vi "Calibration_user_input.vi"(4 "data mode":enum16{"Take new data point", "Refit Curve"}(ring), 6 "Mode":T4, 7 "Fixed n":bool, 8 "OK":T14, 9 "Sampling speeds":T5={"Samples /ch"=300, "Sampling Rate /ch (Hz)"=50.0} {"Sampling Rate /ch (Hz)" min=0 format="%.2f"; "Samples /ch" min=0 step=1}) -> (1 "Sampling speeds Output":T5={"Samples /ch"=300, "Sampling Rate /ch (Hz)"=50.0} {"Sampling Rate /ch (Hz)" min=0 format="%.2f"; "Samples /ch" min=0 step=1}, 2 "Fixed n out":bool, 3 "Temp (deg C)":dbl=21.0 format="%.1f", 5 "Abs Press (mbar)":dbl=1013.0 format="%.1f")   [LabVIEW 2011]
uses:
  Controls/ok_button.ctl
  Controls/Board_Types.ctl
  Controls/Cal_Inst_type.ctl
  Calib_setup.ctl
  Controls/Ref_Inst_type.ctl
  Calib_mode.ctl
  Controls/PWA_Data.ctl
  File/Setup_Filetype.ctl
  Controls/Inst_type.ctl
  ADAM Client/Sub VIs/ADAM Controls/Channel_names.ctl
  Controls/Setup.ctl
  Globals/Calib_global.vi
  Globals/Meas_global.vi
  Globals/LDA_meas_global_1.vi
  Globals/LDA_meas_global_2.vi
panel:
  in  "PWA Data":T1
  in  "Preston tube diammeter in mm":dbl min=0.0
  in  "Reference instrument Orig":T3={"high limit (10V)"=4.0, "low limit (-10V)"=0.0, "Ch No"=4, "Off ch no"=0, "Calib filename"=path "", "Ref Instrument type"=enum."Enter Value"} {"Off ch no" min=0 max=1; "Ch No" min=0 max=7; "low limit (-10V)" min=-10 max=10 format="%.1f"; "high limit (10V)" min=-10 max=10 format="%.1f"}
  out "Message":string
  in  "Ref Instrument type":T2
  out "Info":string
  out "XW Angle Calib Present?":bool
  out "XW Velocity Calib Present?":bool
  in  "Edit temp and Press":bool
  out "2nd ref instrument":T6={"2nd Ref type"=enum."LDA", "2nd inst present"=TRUE}
  in  "Ref vel for angle calib":T7={"high limit (10V)"=6.0, "low limit (-10V)"=0.0, "Ch No"=4, "Off ch no"=0, "Calib filename"=path "", "Ref Instrument type"=enum."LDA"} {"Off ch no" min=0 max=1; "Ch No" min=0 max=50; "low limit (-10V)" min=-10 max=10 format="%.1f"; "high limit (10V)" min=-10 max=10 format="%.1f"}
  out "Instrument type":T8=enum."Cross wire angle"
  in  "angle calib":T9(ring)
  in  "Reference instrument":T7={"high limit (10V)"=4.0, "low limit (-10V)"=0.0, "Ch No"=4, "Off ch no"=0, "Calib filename"=path "", "Ref Instrument type"=enum."Enter Value"} {"Off ch no" min=0 max=1; "Ch No" min=0 max=50; "low limit (-10V)" min=-10 max=10 format="%.1f"; "high limit (10V)" min=-10 max=10 format="%.1f"}
  in  "instrument to calibrate":T10(array[cluster])=[{"high limit (10V)"=5.0, "low limit (-10V)"=3.0, "Ch No"=1, "Off ch no"=1}, {"high limit (10V)"=5.0, "low limit (-10V)"=3.0, "Ch No"=2, "Off ch no"=1}] {"Off ch no" min=0 max=1; "Ch No" min=0 max=50; "low limit (-10V)" min=-10 max=10 format="%.3f"; "high limit (10V)" min=-10 max=10 format="%.3f"}
  in  "Instrument type":T8=enum."Pressure Transducer"
  out "Calib filename":path
  in  "Type":T11={"high limit (10V)"=4.0, "low limit (-10V)"=0.0, "Ch No"=4, "Var name"="LDA"} {"Ch No" min=0 max=7; "low limit (-10V)" min=-10 max=10 format="%.3f"; "high limit (10V)" min=-10 max=10 format="%.3f"}
  in  "Acquisition Method":T12
  out "Ch & spans":T13(array[cluster])=[{"high limit (10V)"=5.0, "low limit (-10V)"=3.0, "Ch No"=1, "Var name"="Cross wire 1"}, {"high limit (10V)"=5.0, "low limit (-10V)"=3.0, "Ch No"=2, "Var name"="Cross wire 2"}] {"Ch No" min=0 max=7; "low limit (-10V)" min=-10 max=10 format="%.3f"; "high limit (10V)" min=-10 max=10 format="%.3f"}
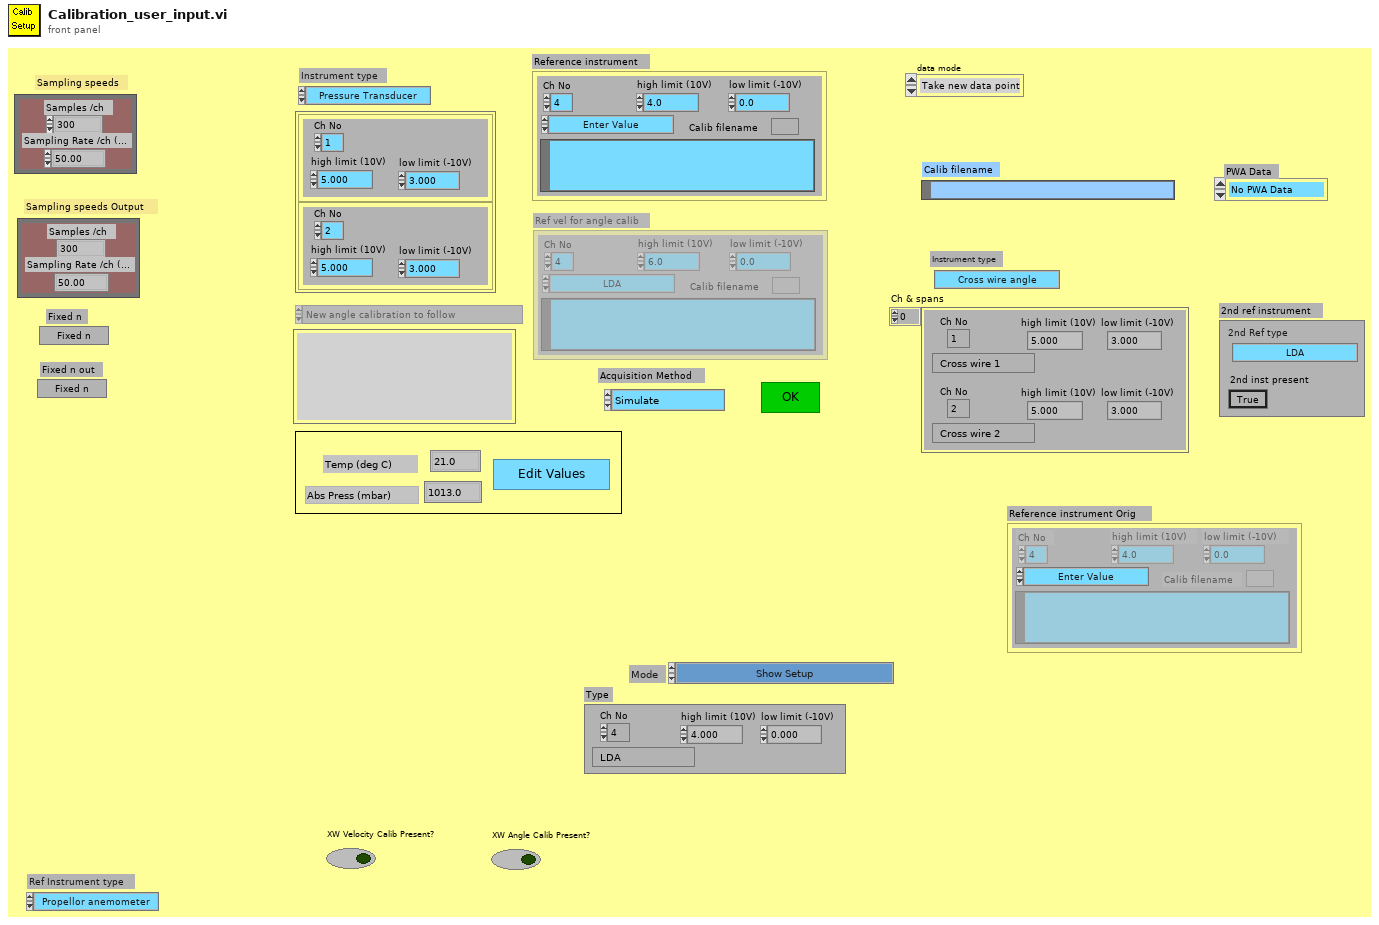
[diagram p1: front panel]
types:
  T1 = typedef "PWA_Data.ctl" = enum16{"No PWA Data", "One Ch PWA"}
  T2 = typedef "Ref_Inst_type.ctl" = enum16{"Propellor anemometer", "Pressure Transducer", "Raw voltage", "Pitot-static tube", "Preston tube", "Generic Linear", "Generic Polynomial", "Thermocouple", "LDA", "Enter Value", "ADAM Channel"}
  T3 = cluster{"high limit (10V)":sgl, "low limit (-10V)":sgl, "Ch No":i16, "Off ch no":i8, "Calib filename":path, "Ref Instrument type":T2}
  T4 = typedef "Calib_mode.ctl" = enum16{"Show Setup", "Take a New Calibration Point", "Refit Curve", "Setup Front Panel"}
  T5 = cluster{"Samples /ch":i32, "Sampling Rate /ch (Hz)":sgl}
  T6 = cluster{"2nd Ref type":T2, "2nd inst present":bool}
  T7 = typedef "Calib_setup.ctl" = cluster{"high limit (10V)":sgl, "low limit (-10V)":sgl, "Ch No":i16, "Off ch no":i8, "Calib filename":path, "Ref Instrument type":T2}
  T8 = typedef "Cal_Inst_type.ctl" = enum16{"Propeller anemometer", "Pressure Transducer", "Hot wire", "Cross wire velocity", "Cross wire angle", "Generic Linear", "Generic Polynomial", "Generic BackPoly", "Fast FID", "Thermocouple", "Cold wire", "Pulsed Wire"}
  T9 = enum16{"New angle calibration to follow", "Use the most recent angle calibration"}
  T10 = cluster{"high limit (10V)":sgl, "low limit (-10V)":sgl, "Ch No":i16, "Off ch no":i8}[]
  T11 = cluster{"high limit (10V)":sgl, "low limit (-10V)":sgl, "Ch No":i16, "Var name":string}
  T12 = typedef "Board_Types.ctl" = enum16{"Simulate", "Local ADAM", "Server ADAM", "NI-DAQmx", "NI-DAQmxBase", "ADC488", "DT LV-link"}
  T13 = cluster{"high limit (10V)":sgl, "low limit (-10V)":sgl, "Ch No":i16, "Var name":string}[]
  T14 = typedef "ok_button.ctl" = bool
  T15 = typedef "Setup_Filetype.ctl" = enum16{"Measurement Setups", "Calibration Setups", "General", "Results File Plotter Setups", "Speed Calib Tweaks"}
  T16 = typedef "Inst_type.ctl" = enum16{"Propeller anemometer", "Raw voltage", "Pressure Transducer", "Pitot-static tube", "Preston tube", "Hot wire", "Cross wire 1", "Cross wire 2", "Generic Linear", "Generic Polynomial", "Generic BackPoly", "Fast FID", "Thermocouple", "Cold wire", "Pulsed Wire", "LDA Vel", "LDA Tran time", "LDA Arr time"}
  T17 = typedef "Channel_names.ctl" = enum16{"Active Only", "Active + Off", "All Channels"}
  T18 = typedef "Setup.ctl" = enum16{"Run Program", "Show Setup", "Save Current Setup", "Setup Front Panel"}
  T19 = cluster{"high limit (10V)":sgl, "low limit (-10V)":sgl, "Ch No":i16, "Off ch no":i8}
  T20 = typedef "BSA_Type.ctl" = enum16{"57N11", "BSA F60"}
  T21 = typedef "BSA_info_Cluster.ctl" = cluster{"GPIB Address":string, "No of Check Bytes":i32, "Extra Info":string, "COLOUR":u32, "Wavelength (nm)":dbl}
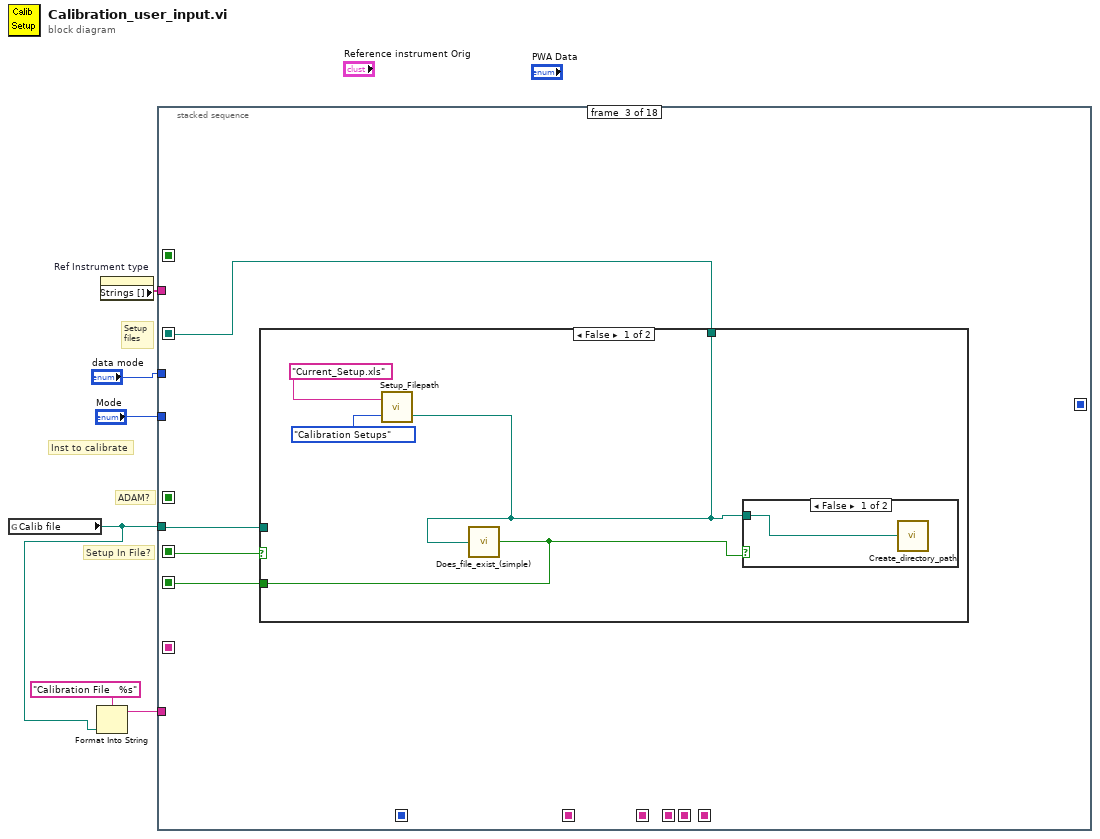
[diagram p0: block diagram]
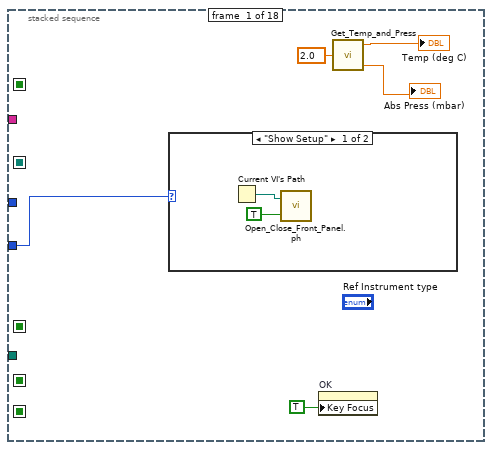
[diagram p2: hidden frame]
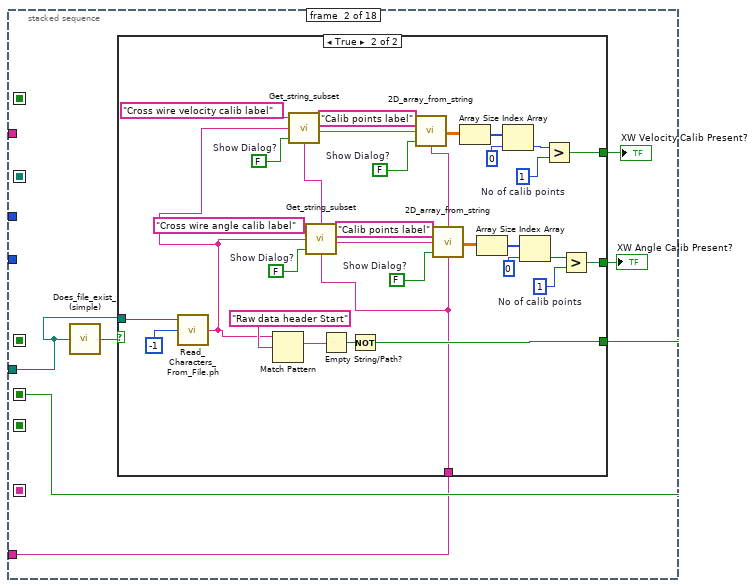
[diagram p4: hidden frame]
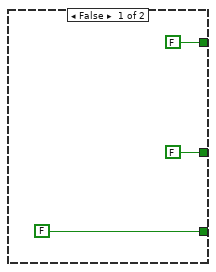
[diagram p5: hidden frame]
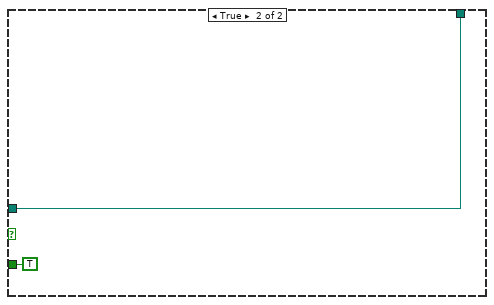
[diagram p7: hidden frame]
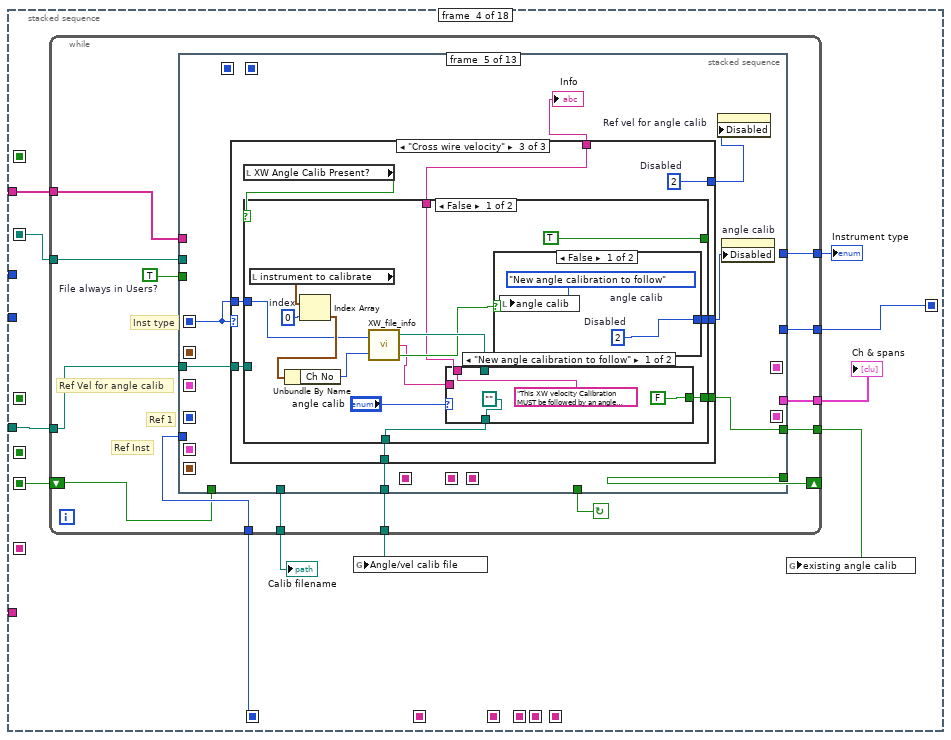
[diagram p8: hidden frame]
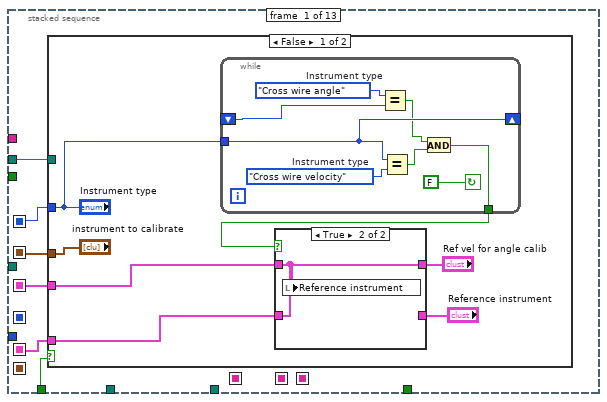
[diagram p9: hidden frame]
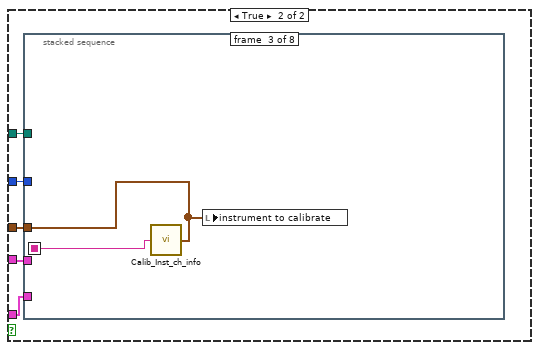
[diagram p11: hidden frame]
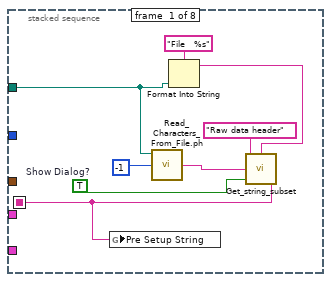
[diagram p12: hidden frame]
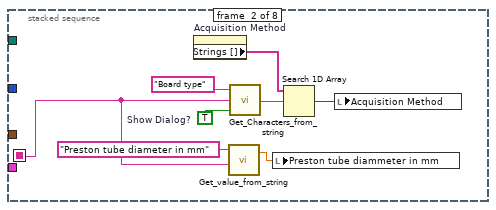
[diagram p13: hidden frame]
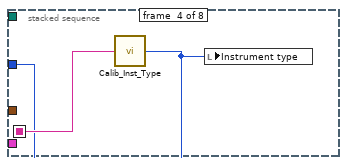
[diagram p14: hidden frame]
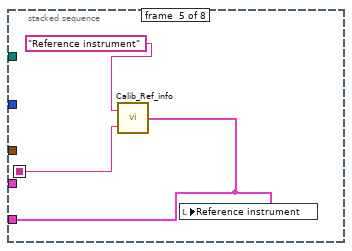
[diagram p15: hidden frame]
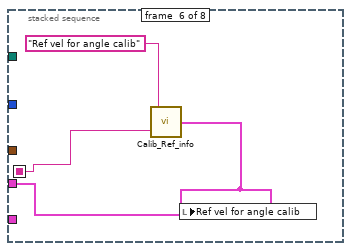
[diagram p16: hidden frame]
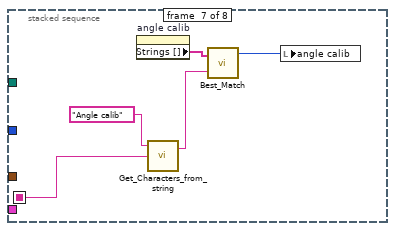
[diagram p17: hidden frame]
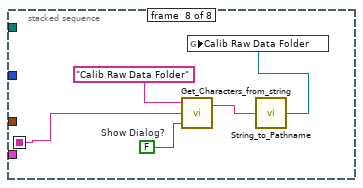
[diagram p18: hidden frame]
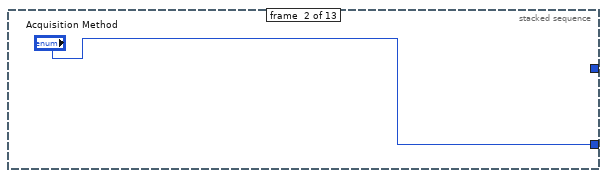
[diagram p19: hidden frame]
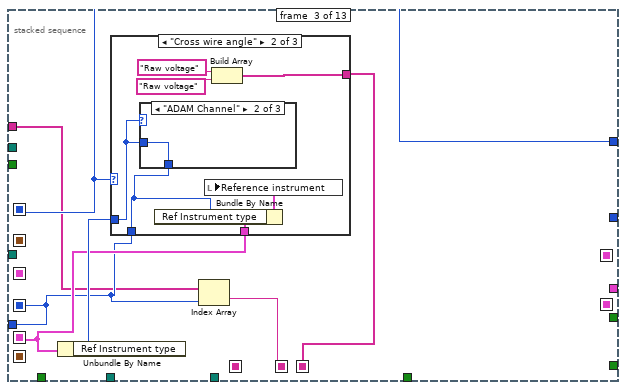
[diagram p20: hidden frame]
diagram:
  # "Inst to calibrate"
  # "Setup In File?"
  # "Setup\nfiles"
  # "ADAM?"
  n1 = global read "Calib_global.vi" "Calib file"() -> (w2:path)
  n2 = Format Into String(format string="Calibration File   %s", w2) -> (resulting string=w1:string)  [unwired: 2 in, 1 out]
  n3 = property on="Ref Instrument type" class="Enum (strict)"() -> ("Strings []"=w4:string[])  [unwired: 2 in, 2 out]
  n4 = stacked-sequence {
    seq-local: [_ _ w55 _ _ _ _ _ _ _ _ _ _ _ _ _ _ _] -> [_ _ _ w72 _ _ _ _ _ _ _ _ _ _ _ _ _ _]
    seq-local: [_ _ w56 _ _ _ _ _ _ _ _ _ _ _ _ _ _ _] -> [_ _ _ w70 _ _ _ _ _ _ _ _ _ _ _ _ _ _]
    seq-local: [_ _ _ w69 _ _ _ _ _ _ _ _ _ _ _ _ _ _] -> [_ _ _ _ _ _ _ w603 _ _ _ _ _ _ _ _ _ _]
    seq-local: [_ _ _ _ _ _ _ w604 _ _ _ _ _ _ _ _ _ _] -> [_ _ _ _ _ _ _ _ w621 _ _ _ _ _ _ _ _ _]
    seq-local: [_ _ _ _ _ _ _ _ w624 _ _ _ _ _ _ _ _ _] -> [_ _ _ _ _ _ _ _ _ _ _ _ _ _ w801 _ _ _]
    seq-local: [_ _ _ w68 _ _ _ _ _ _ _ _ _ _ _ _ _ _] -> [_ _ _ _ _ _ _ _ _ _ w716 _ _ _ _ _ _ _]
    seq-local: [_ _ _ _ _ _ _ _ _ _ w713 _ _ _ _ _ _ _] -> [_ _ _ _ _ _ _ _ _ _ _ _ _ _ w800 _ w835 _]
    seq-local: [_ _ _ _ _ _ _ _ _ _ w710 _ _ _ _ _ _ _] -> [_ _ _ _ _ _ _ _ _ _ _ _ _ _ _ w807 _ _]
    seq-local: [_ w19 _ _ _ _ _ _ _ _ _ _ _ _ _ _ _ _] -> [_ _ w54 _ _ _ _ _ _ _ _ _ _ _ _ _ _ _]
    seq-local: [_ _ _ _ _ _ _ _ _ _ _ w726 _ _ _ _ _ _] -> [_ _ _ _ _ _ _ _ _ _ _ _ _ _ w793 _ _ _]
    seq-local: [_ _ _ _ _ _ _ _ _ _ _ _ _ w751 _ _ _ _] -> [_ _ _ _ _ _ _ _ _ _ _ _ _ _ w781 _ _ _]
    seq-local: [_ _ _ _ _ _ _ _ _ _ _ _ w733 _ _ _ _ _] -> [_ _ _ _ _ _ _ _ _ _ _ _ _ _ w777 _ w825 _]
    seq-local: [_ _ _ _ _ _ _ _ _ w659 _ _ _ _ _ _ _ _] -> [_ _ _ _ _ _ _ _ _ _ _ _ _ _ w776 _ _ _]
    tunnel: "Mode" -> [w7 _ _ _ w526 w544 _ _ w623 w672 _ _ w734 _ _ w809 _ w852]
    tunnel: "data mode" -> [_ _ _ _ w520 _ _ _ _ _ _ _ _ _ _ _ _ _]
    tunnel: w2 -> [_ w17 w53 w65 _ _ _ _ _ _ _ _ _ _ _ _ _ _]
    tunnel: w4 -> [_ _ _ w64 _ _ _ _ _ _ _ _ _ _ _ _ _ _]
    tunnel: w1 -> [_ w14 _ _ _ _ _ _ _ _ _ _ _ _ _ _ _ _]
    frame #0 {
      n5 = case shown="\"Show Setup\"" w7 {
        frame "Show Setup" {
          n6 = Current VI's Path() -> (path=w13:path)
          n7 = call "Open_Close_Front_Panel.ph.vi"("Front Panel Window:Open"=TRUE, "VI path"=w13) -> ()  [unwired: 2 out]
        }
        frame "Take a New Calibration Point", Default {
        }
      }
      n8 = property on="OK" class="Bool"("Key Focus"=TRUE) -> ()  [unwired: 2 in, 2 out]
      n9 = call "Get_Temp_and_Press.vi"("Averaging time (mins)"=2.0) -> ("Abs Press (mbar)"=→"Abs Press (mbar)":dbl, "Temperature"=→"Temp (deg C)":dbl)  [unwired: 3 out]
    }
    frame #1 {
      n10 = call "Does_file_exist_(simple).vi"("Pathname"=w17) -> ("exists?"=w18:bool)
      n11 = case shown="True" w18 {
        tunnel: [FALSE w48] -> w19
        tunnel: w17 -> [_ w47]
        tunnel: [FALSE w25] -> w16
        tunnel: [FALSE w24] -> w15
        tunnel: w14 -> [_ w23]
        frame False {
        }
        frame True {
          w36 = 1  # No of calib points
          w30 = FALSE  # Show Dialog?
          w28 = FALSE  # Show Dialog?
          w37 = 1  # No of calib points
          w43 = FALSE  # Show Dialog?
          w45 = FALSE  # Show Dialog?
          n12 = call "Read_Characters_From_File.ph.vi"("file path (dialog if empty)"=w47, "number of characters (all:-1)"=-1) -> ("character string"=w26:string)  [unwired: 7 out]
          n13 = Match Pattern(string=w26, regular expression="Raw data header Start") -> (match substring=w50:string)  [unwired: 4 out]
          n14 = call "Get_string_subset.vi"("String Name"=w23, "Show Dialog?"=w28, "String to split"=w26, "File Label"="Cross wire velocity calib label") -> ("Output string"=w34:string)  [unwired: 1 out]
          n15 = call "Get_string_subset.vi"("String Name"=w23, "Show Dialog?"=w45, "String to split"=w26, "File Label"="Cross wire angle calib label") -> ("Output string"=w39:string)  [unwired: 1 out]
          n16 = Empty String/Path?(string/path=w50) -> (empty?=w49:bool)
          n17 = Not(x=w49) -> (.not. x?=w48:bool)
          n18 = call "2D_array_from_string.vi"("String Name"=w23, "Show Dialog?"=w30, "Input string"=w34, "Array title"="Calib points label") -> ("2D data array"=w31:dbl[][])
          n19 = call "2D_array_from_string.vi"("String Name"=w23, "Show Dialog?"=w43, "Input string"=w39, "Array title"="Calib points label") -> ("2D data array"=w42:dbl[][])
          n20 = Array Size(array=w31) -> (size(s)=w32:i32[])
          n21 = Array Size(array=w42) -> (size(s)=w41:i32[])
          n22 = Index Array(array=w32, index=0 ("Index")) -> (element=w35:i32)
          n23 = Index Array(array=w41, index=0 ("Index")) -> (element=w38:i32)
          n24 = Greater?(x=w35, y=w36) -> (0:w24:bool)
          n25 = Greater?(x=w38, y=w37) -> (0:w25:bool)
        }
      }
      "XW Velocity Calib Present?" <- w15
      "XW Angle Calib Present?" <- w16
    }
    frame #2 {
      n26 = case shown="False" w54 {
        tunnel: [w60 TRUE ("exists")] -> w56
        tunnel: [w57 w63] -> w55
        tunnel: w53 -> [_ w63]
        frame False {
          n27 = call "Setup_Filepath.vi"("Setup File Type"=Setup_Filetype."Calibration Setups", "Filename in"="Current_Setup.xls") -> ("Filename Out"=w57:path)  [unwired: 1 out]
          n28 = call "Does_file_exist_(simple).vi"("Pathname"=w57) -> ("exists?"=w60:bool)
          n29 = case shown="False" w60 {
            tunnel: w57 -> [w61 _]
            frame False {
              n30 = call "Create_directory_path.vi"("Path name"=w61) -> ()  [unwired: 1 in, 2 out]
            }
            frame True {
            }
          }
        }
        frame True {
        }
      }
    }
    frame #3 {
      n31 = while {
        tunnel: w64 -> [w78]
        shift-left: w70 -> [w81]
        shift-right: [w80] -> _
        tunnel: [w82] -> w71
        tunnel: w72 -> [w83]
        tunnel: [w84] -> w67
        tunnel: [w85] -> w74
        tunnel: [w86] -> w69
        tunnel: [w87] -> w73
        tunnel: [w88] -> w68
        tunnel: [w76] -> w66
        tunnel: w65 -> [w75]
        stop <- w79 continue-if-true
        w77 = TRUE  # File always in Users?
        # "Ref 1"
        # "Ref Inst"
        # "Ref Vel for angle calib"
        # "Inst type"
        n32 = stacked-sequence {
          seq-local: [_ _ w157 _ _ _ _ _ _ _ _ _ _] -> [_ _ _ _ _ w273 _ _ _ _ _ _ _]
          seq-local: [_ _ w161 _ _ _ _ _ _ _ _ _ _] -> [_ _ _ _ _ _ _ _ w424 _ _ _ _]
          seq-local: [_ _ _ _ _ w267 _ _ _ _ _ _ _] -> [_ _ _ _ _ _ _ _ _ w441 _ _ _]
          seq-local: [_ _ w156 _ _ _ _ _ _ _ _ _ _] -> [_ _ _ _ _ _ _ _ _ w439 _ _ _]
          seq-local: [_ _ _ _ _ _ _ _ w423 _ _ _ _] -> [_ _ _ _ _ _ _ _ _ w440 _ _ _]
          seq-local: [_ _ _ _ _ _ _ w345 _ _ _ _ _] -> [_ _ _ _ _ _ _ _ _ w436 _ _ _]
          seq-local: [_ _ _ _ _ _ w341 _ _ _ _ _ _] -> [_ _ _ _ _ _ _ _ _ w435 _ _ _]
          seq-local: [w92 _ _ _ _ _ _ _ _ _ _ _ _] -> [_ _ w159 w184 w197 _ _ w346 _ _ _ _ _]
          seq-local: [w91 _ _ _ _ _ _ _ _ _ _ _ _] -> [_ _ _ w183 _ _ _ _ _ _ _ _ _]
          seq-local: [w90 _ _ _ _ _ _ _ _ _ _ _ _] -> [_ _ _ _ _ _ w343 w347 _ w434 _ _ _]
          seq-local: [w89 _ _ _ _ _ _ _ _ _ _ _ _] -> [_ _ w158 _ _ _ _ _ _ w433 _ _ w519]
          seq-local: [_ _ _ _ _ _ _ _ _ w432 _ _ _] -> [_ _ _ _ _ _ _ _ _ _ _ w478 _]
          seq-local: [_ _ _ w179 _ _ _ _ _ _ _ _ _] -> [_ _ _ _ _ _ _ _ w422 _ _ _ _]
          tunnel: [_ "Acquisition Method" _ _ _ _ _ _ _ _ _ _ _] -> w88
          tunnel: [_ _ _ _ _ _ _ _ _ w438 _ _ _] -> w87
          tunnel: [_ _ w157 _ _ _ _ _ _ _ _ _ _] -> w86
          tunnel: [_ _ _ _ _ _ _ _ _ w432 _ _ _] -> w85
          tunnel: [_ _ _ _ w202 _ _ _ _ _ _ _ _] -> w84
          tunnel: w83 -> [w94 _ _ _ _ _ _ _ _ _ _ _ _]
          tunnel: [_ _ w159 _ _ _ _ _ _ _ _ _ _] -> w82
          tunnel: w81 -> [w93 _ _ _ _ _ _ _ _ _ _ _ _]
          tunnel: [_ _ _ _ _ _ _ _ _ _ _ FALSE _] -> w80
          tunnel: [_ _ _ _ _ _ _ _ _ _ _ w476 _] -> w79
          tunnel: w78 -> [_ _ w155 _ _ _ w340 _ _ _ _ _ _]
          tunnel: w77 -> [_ _ _ _ _ _ _ _ _ _ _ _ _]
          tunnel: [_ _ _ _ w201 _ _ _ _ _ _ _ _] -> w76
          tunnel: w75 -> [_ _ _ _ w203 _ _ _ _ _ _ _ _]
          frame #0 {
            n33 = case shown="False" w93 {
              tunnel: w94 -> [_ w117]
              tunnel: ["Instrument type" w115] -> w92
              tunnel: ["instrument to calibrate" w116] -> w91
              tunnel: [w96 w113] -> w90
              tunnel: [w98 w114] -> w89
              frame False {
                n34 = while {
                  shift-right: [w110] -> _
                  shift-left: _ -> [w108]
                  tunnel: "Instrument type" -> [w110]
                  tunnel: [w105] -> w99
                  stop <- FALSE continue-if-true
                  w109 = Cal_Inst_type."Cross wire angle"  # Instrument type
                  w111 = Cal_Inst_type."Cross wire velocity"  # Instrument type
                  n35 = Equal?(x=w109, y=w108) -> (x = y?=w106:bool)
                  n36 = Equal?(x=w110, y=w111) -> (x = y?=w107:bool)
                  n37 = And(x=w106, y=w107) -> (x .and. y?=w105:bool)
                }
                n38 = case shown="True" w99 {
                  tunnel: [w103 w104] -> w98
                  tunnel: "Reference instrument" -> [w103 _]
                  tunnel: [w102 w104] -> w96
                  tunnel: "Ref vel for angle calib" -> [w102 w104]
                  frame False {
                  }
                  frame True {
                    n39 = local write "Reference instrument"(w104) -> ()
                  }
                }
              }
              frame True {
                n40 = stacked-sequence {
                  seq-local: [w122 _ _ _ _ _ _ _] -> [_ w128 w135 w137 w139 w142 w146 w151]
                  tunnel: w117 -> [w119 _ _ _ _ _ _ _]
                  tunnel: [_ _ w134 _ _ _ _ _] -> w116
                  tunnel: [_ _ _ w136 _ _ _ _] -> w115
                  tunnel: [_ _ _ _ w138 _ _ _] -> w114
                  tunnel: [_ _ _ _ _ w141 _ _] -> w113
                  frame #0 {
                    w121 = TRUE  # Show Dialog?
                    n41 = call "Read_Characters_From_File.ph.vi"("file path (dialog if empty)"=w119, "number of characters (all:-1)"=-1) -> ("character string"=w125:string)  [unwired: 7 out]
                    n42 = Format Into String(format string="File   %s", w119) -> (resulting string=w118:string)  [unwired: 2 in, 1 out]
                    n43 = call "Get_string_subset.vi"("String Name"=w118, "Show Dialog?"=w121, "String to split"=w125, "File Label"="Raw data header") -> ("Output string"=w122:string)  [unwired: 1 out]
                    n44 = global write "Calib_global.vi" "Pre Setup String"(w122) -> ()
                  }
                  frame #1 {
                    w133 = TRUE  # Show Dialog?
                    n45 = property on="Acquisition Method" class="Enum (strict)"() -> ("Strings []"=w129:string[])  [unwired: 2 in, 2 out]
                    n46 = call "Get_value_from_string.vi"("Input string"=w128, "Variable name"="Preston tube diameter in mm") -> ("Value"=w126:dbl)  [unwired: 1 in, 1 out]
                    n47 = call "Get_Characters_from_string.vi"("Show Dialog?"=w133, "Input string"=w128, "Variable name"="Board type") -> ("Value"=w131:string)  [unwired: 1 out]
                    n48 = local write "Preston tube diammeter in mm"(w126) -> ()
                    n49 = Search 1D Array(1D array=w129, element=w131) -> (index of element=w130:i32)  [unwired: 1 out]
                    n50 = local write "Acquisition Method"(w130) -> ()
                  }
                  frame #2 {
                    n51 = call "Calib_Inst_ch_info.vi"("Input string"=w135) -> ("instrument to calibrate"=w134:T10)
                    n52 = local write "instrument to calibrate"(w134) -> ()
                  }
                  frame #3 {
                    n53 = call "Calib_Inst_Type.vi"("Input string"=w137) -> ("Instrument type"=w136:T8)
                    n54 = local write "Instrument type"(w136) -> ()
                  }
                  frame #4 {
                    n55 = call "Calib_Ref_info.vi"("Input string"=w139, "Reference Name"="Reference instrument") -> ("Reference instrument"=w138:T7)
                    n56 = local write "Reference instrument"(w138) -> ()
                  }
                  frame #5 {
                    n57 = call "Calib_Ref_info.vi"("Input string"=w142, "Reference Name"="Ref vel for angle calib") -> ("Reference instrument"=w141:T7)
                    n58 = local write "Ref vel for angle calib"(w141) -> ()
                  }
                  frame #6 {
                    n59 = property on="angle calib" class="Enum (strict)"() -> ("Strings []"=w148:string[])  [unwired: 2 in, 2 out]
                    n60 = call "Get_Characters_from_string.vi"("Input string"=w146, "Variable name"="Angle calib") -> ("Value"=w145:string)  [unwired: 1 in, 1 out]
                    n61 = call "Best_Match.vi"("Input String"=w145, "String Options"=w148) -> ("index of element"=w144:i32)  [unwired: 1 out]
                    n62 = local write "angle calib"(w144) -> ()
                  }
                  frame #7 {
                    w152 = FALSE  # Show Dialog?
                    n63 = call "Get_Characters_from_string.vi"("Show Dialog?"=w152, "Input string"=w151, "Variable name"="Calib Raw Data Folder") -> ("Value"=w150:string)  [unwired: 1 out]
                    n64 = call "String_to_Pathname.vi"("Input String"=w150) -> ("path"=w149:path)
                    n65 = global write "Calib_global.vi" "Calib Raw Data Folder"(w149) -> ()
                  }
                }
              }
            }
          }
          frame #1 {
          }
          frame #2 {
            n66 = Unbundle By Name(w158) -> ("Ref Instrument type"=w160:T2)
            n67 = case shown="\"Cross wire angle\"" w159 {
              tunnel: [w164 w172 w177] -> w161
              tunnel: w160 -> [w162 w166 w176]
              tunnel: [w162 w169 w176] -> w157
              tunnel: w158 -> [_ w170 _]
              frame "Cross wire velocity" {
                n68 = Build Array("Raw voltage", "Raw voltage") -> (w164:string[])
              }
              frame "Cross wire angle" {
                n69 = case shown="\"ADAM Channel\"" w166 {
                  tunnel: [w173 w174 Ref_Inst_type."Enter Value" ("Ref Instrument type")] -> w169
                  tunnel: w166 -> [w173 w174 _]
                  frame "Enter Value" {
                  }
                  frame "ADAM Channel" {
                  }
                  frame "LDA", Default {
                  }
                }
                n70 = Bundle By Name(cluster=w170, "Ref Instrument type"=w169) -> (w171:T7)
                n71 = local write "Reference instrument"(w171) -> ()
                n72 = Build Array("Raw voltage", "Raw voltage") -> (w172:string[])
              }
              frame "Generic Linear", Default {
                n73 = Build Array("Raw voltage") -> (w177:string[])
              }
            }
            n74 = Index Array(array=w155, index=w157) -> (element=w156:string)
          }
          frame #3 {
            n75 = Array Size(array=w183) -> (size(s)=w182:i32)
            n76 = case shown="\"Pulsed Wire\"" w184 {
              tunnel: [2 2 1 0] -> w181
              frame "Cross wire velocity" {
              }
              frame "Cross wire angle" {
              }
              frame "Generic Linear", Default {
              }
              frame "Pulsed Wire" {
              }
            }
            n77 = Equal?(x=w181, y=w182) -> (x = y?=w180:bool)
            n78 = case shown="False" w180 {
              tunnel: w181 -> [w190 _]
              tunnel: w183 -> [w186 w192]
              tunnel: [w185 w192] -> w179
              frame False {
                n79 = Index Array(array=w186, index=0) -> (element=w187:T19)
                n80 = Build Array (concatenate)(w186, w187) -> (w189:T10)
                n81 = for {
                  N: w190 -> [_]
                  tunnel: w189 -> [w191] mode=indexing
                  tunnel: [w191] -> w185 mode=indexing
                }
                n82 = local write "instrument to calibrate"(w185) -> ()
              }
              frame True {
              }
            }
          }
          frame #4 {
            n83 = case shown="\"Cross wire velocity\"" w197 {
              tunnel: w203 -> [_ w214 w236]
              tunnel: [path "" w215 w237] -> w202
              tunnel: [FALSE w213 w235] -> w201
              tunnel: [w204 w209 w231] -> w200
              tunnel: [w206 w212 w234] -> w199
              tunnel: ["" w211 w232] -> w198
              tunnel: w197 -> [_ w210 w233]
              frame "Propeller anemometer", Default {
                w204 = u8 2  # Disabled
                w206 = u8 2  # Disabled
              }
              frame "Cross wire angle" {
                w209 = u8 0  # Disabled
                w212 = u8 2  # Disabled
                n84 = local read "XW Velocity Calib Present?"() -> (w216:bool)
                n85 = case shown="False" w216 {
                  tunnel: [w220 w230] -> w215
                  tunnel: w214 -> [_ w230]
                  tunnel: [TRUE TRUE] -> w213
                  tunnel: [w218 w228] -> w211
                  tunnel: w210 -> [w217 _]
                  frame False {
                    w224 = 0  # index
                    n86 = local read "instrument to calibrate"() -> (w225:T10)
                    n87 = Index Array(array=w225, index=w224) -> (element=w223:T19)
                    n88 = Unbundle By Name(w223) -> ("Ch No"=w221:i16)
                    n89 = call "XW_file_info.vi"("Instrument type"=w217, "Ch No"=w221) -> ("Filename"=w220:path, "resulting string"=w218:string, "File Exists?"=w219:bool)
                    n90 = case shown="False" w219 {
                      frame False {
                        w226 = Cal_Inst_type."Cross wire velocity"  # Instrument type
                        w227 = "You need to do a velocity calibration before you can do the angle calibration"  # message
                        n91 = local write "Instrument type"(w226) -> ()
                        n92 = One Button Dialog(message=w227) -> ()  [unwired: 2 out]
                      }
                      frame True {
                      }
                    }
                  }
                  frame True {
                    w228 = "Will use the velocity Calibration info already in the Calibration file. "  # resulting string
                  }
                }
              }
              frame "Cross wire velocity" {
                w231 = u8 2  # Disabled
                n93 = local read "XW Angle Calib Present?"() -> (w238:bool)
                n94 = case shown="False" w238 {
                  tunnel: [w247 w266] -> w237
                  tunnel: w236 -> [_ w266]
                  tunnel: [TRUE FALSE] -> _
                  tunnel: [w246 TRUE] -> w235
                  tunnel: [w245 w263] -> w234
                  tunnel: w233 -> [w243 _]
                  tunnel: [w240 w262] -> w232
                  frame False {
                    w251 = 0  # index
                    n95 = local read "instrument to calibrate"() -> (w252:T10)
                    n96 = Index Array(array=w252, index=w251) -> (element=w250:T19)
                    n97 = Unbundle By Name(w250) -> ("Ch No"=w244:i16)
                    n98 = call "XW_file_info.vi"("Instrument type"=w243, "Ch No"=w244) -> ("Filename"=w242:path, "resulting string"=w239:string, "File Exists?"=w241:bool)
                    n99 = case shown="\"New angle calibration to follow\"" "angle calib" {
                      tunnel: [path "" w258] -> w247
                      tunnel: w242 -> [_ w258]
                      tunnel: [FALSE TRUE] -> w246
                      tunnel: ["This XW velocity Calibration MUST be followed by an angle calibration, before XW measurements can be made." w256] -> w240
                      tunnel: w239 -> [_ w256]
                      frame "New angle calibration to follow" {
                      }
                      frame "Use the most recent angle calibration" {
                      }
                    }
                    n100 = case shown="False" w241 {
                      tunnel: [w259 w261] -> w245
                      frame False {
                        w259 = u8 2  # Disabled
                        w260 = T9."New angle calibration to follow"  # angle calib
                        n101 = local write "angle calib"(w260) -> ()
                      }
                      frame True {
                        w261 = u8 0  # Disabled
                      }
                    }
                  }
                  frame True {
                    w262 = "Will use the angle Calibration info already in the Calibration file. "  # resulting string
                    w263 = u8 0  # Disabled
                  }
                }
              }
            }
            "Info" <- w198
            n102 = property on="Ref vel for angle calib" class="Clust (strict)"("Disabled"=w200) -> ()  [unwired: 2 in, 2 out]
            n103 = property on="angle calib" class="Enum (strict)"("Disabled"=w199) -> ()  [unwired: 2 in, 2 out]
          }
          frame #5 {
            n104 = case shown="\"Generic Polynomial\"" w273 {
              tunnel: [u8 0 u8 0 u8 0 u8 0 u8 0 u8 0 u8 0 u8 2 u8 2 u8 2 u8 2] -> w268
              tunnel: [u8 0 u8 0 u8 2 u8 0 u8 0 u8 0 u8 0 u8 2 u8 2 u8 2 u8 2] -> w272
              tunnel: [u8 0 u8 0 u8 0 u8 0 u8 0 u8 0 u8 0 u8 2 u8 2 u8 2 u8 2] -> w271
              tunnel: [u8 0 u8 0 u8 0 u8 0 u8 0 u8 0 u8 0 u8 2 u8 2 u8 2 u8 2] -> w270
              tunnel: [u8 0 u8 0 u8 0 u8 0 u8 0 u8 0 u8 0 u8 2 u8 2 u8 2 u8 2] -> w269
              tunnel: [1 1 1 1 1 1 1 0 0 0 0] -> w267
              frame "Propellor anemometer" {
              }
              frame "Pressure Transducer" {
              }
              frame "Raw voltage" {
              }
              frame "Pitot-static tube" {
              }
              frame "Preston tube" {
              }
              frame "Generic Linear" {
              }
              frame "Generic Polynomial" {
              }
              frame "Thermocouple" {
              }
              frame "LDA" {
              }
              frame "Enter Value" {
              }
              frame "ADAM Channel" {
              }
            }
            n105 = property on="Calib filename" class="Path"("Disabled"=w272) -> ()  [unwired: 2 in, 2 out]
            n106 = property on="Ch No" class="DigNum (strict)"("Disabled"=w271) -> ()  [unwired: 2 in, 2 out]
            n107 = property on="high limit (10V)" class="DigNum (strict)"("Disabled"=w270) -> ()  [unwired: 2 in, 2 out]
            n108 = property on="low limit (-10V)" class="DigNum (strict)"("Disabled"=w269) -> ()  [unwired: 2 in, 2 out]
            n109 = property on="Off ch no" class="DigNum (strict)"("Disabled"=w268) -> ()  [unwired: 2 in, 2 out]
          }
          frame #6 {
            n110 = Unbundle By Name(w343) -> ("Ref Instrument type"=w342:T2)
            n111 = Index Array(array=w340, index=w342) -> (element=w341:string)
          }
          frame #7 {
            n112 = Unbundle By Name(w347) -> ("Ref Instrument type"=w348:T2)
            n113 = case shown="\"Generic Polynomial\"" w348 {
              tunnel: [u8 0 u8 0 u8 0 u8 0 u8 0 u8 0 u8 0 u8 0 u8 2 u8 2 u8 2] -> w349
              tunnel: [u8 0 u8 0 u8 2 u8 0 u8 0 u8 0 u8 0 u8 0 u8 2 u8 2 u8 2] -> w353
              tunnel: [u8 0 u8 0 u8 0 u8 0 u8 0 u8 0 u8 0 u8 0 u8 2 u8 2 u8 2] -> w352
              tunnel: [u8 0 u8 0 u8 0 u8 0 u8 0 u8 0 u8 0 u8 0 u8 2 u8 2 u8 2] -> w351
              tunnel: [u8 0 u8 0 u8 0 u8 0 u8 0 u8 0 u8 0 u8 0 u8 2 u8 2 u8 2] -> w350
              tunnel: [enum16{"No 2nd ref inst", "Add 2nd ref inst"}."Add 2nd ref inst" enum16{"No 2nd ref inst", "Add 2nd ref inst"}."Add 2nd ref inst" enum16{"No 2nd ref inst", "Add 2nd ref inst"}."Add 2nd ref inst" enum16{"No 2nd ref inst", "Add 2nd ref inst"}."Add 2nd ref inst" enum16{"No 2nd ref inst", "Add 2nd ref inst"}."Add 2nd ref inst" enum16{"No 2nd ref inst", "Add 2nd ref inst"}."Add 2nd ref inst" enum16{"No 2nd ref inst", "Add 2nd ref inst"}."Add 2nd ref inst" enum16{"No 2nd ref inst", "Add 2nd ref inst"}."Add 2nd ref inst" enum16{"No 2nd ref inst", "Add 2nd ref inst"}."No 2nd ref inst" enum16{"No 2nd ref inst", "Add 2nd ref inst"}."No 2nd ref inst" enum16{"No 2nd ref inst", "Add 2nd ref inst"}."No 2nd ref inst"] -> w344
              frame "Propellor anemometer" {
              }
              frame "Pressure Transducer" {
              }
              frame "Raw voltage" {
              }
              frame "Pitot-static tube" {
              }
              frame "Preston tube" {
              }
              frame "Generic Linear" {
              }
              frame "Generic Polynomial" {
              }
              frame "Thermocouple" {
              }
              frame "LDA" {
              }
              frame "Enter Value" {
              }
              frame "ADAM Channel" {
              }
            }
            n114 = case shown="\"Generic Linear\", Default" w346 {
              tunnel: [w354 enum16{"No 2nd ref inst", "Add 2nd ref inst"}."No 2nd ref inst"] -> w345
              tunnel: w344 -> [w354 _]
              frame "Cross wire angle" {
              }
              frame "Generic Linear", Default {
              }
            }
            n115 = property on="Calib filename" class="Path"("Disabled"=w353) -> ()  [unwired: 2 in, 2 out]
            n116 = property on="low limit (-10V)" class="DigNum (strict)"("Disabled"=w352) -> ()  [unwired: 2 in, 2 out]
            n117 = property on="high limit (10V)" class="DigNum (strict)"("Disabled"=w351) -> ()  [unwired: 2 in, 2 out]
            n118 = property on="Ch No" class="DigNum (strict)"("Disabled"=w350) -> ()  [unwired: 2 in, 2 out]
            n119 = property on="Off ch no" class="DigNum (strict)"("Disabled"=w349) -> ()  [unwired: 2 in, 2 out]
          }
          frame #8 {
            n120 = for {
              tunnel: w424 -> [w431] mode=indexing
              tunnel: [w429] -> w423 mode=indexing
              tunnel: w422 -> [w425] mode=indexing
              n121 = Unbundle By Name(w425) -> ("high limit (10V)"=w428:sgl, "low limit (-10V)"=w427:sgl, "Ch No"=w426:i16)
              n122 = Bundle By Name(cluster="Type", "high limit (10V)"=w428, "low limit (-10V)"=w427, "Ch No"=w426, "Var name"=w431) -> (w429:T11)
            }
          }
          frame #9 {
            n123 = local read "Type"() -> (w437:T11)
            n124 = case shown="..0" w441 {
              tunnel: [w445 w467] -> w432
              tunnel: w440 -> [w448 w461]
              tunnel: w433 -> [_ w464]
              tunnel: w439 -> [_ w463]
              tunnel: [w447 w466] -> w438
              tunnel: w437 -> [w446 w465]
              tunnel: w434 -> [w442 _]
              tunnel: w436 -> [w444 _]
              tunnel: w435 -> [w443 _]
              frame ..0 {
                n125 = case shown="\"No 2nd ref inst\"" w444 {
                  tunnel: [w450 w460] -> w445
                  tunnel: w443 -> [_ w459]
                  tunnel: w442 -> [_ w458]
                  tunnel: w446 -> [_ w457]
                  tunnel: [path "" w456] -> w447
                  tunnel: w448 -> [w450 w451]
                  frame "No 2nd ref inst" {
                  }
                  frame "Add 2nd ref inst" {
                    n126 = Unbundle By Name(w458) -> ("high limit (10V)"=w453:sgl, "low limit (-10V)"=w454:sgl, "Ch No"=w455:i16, "Calib filename"=w456:path)
                    n127 = Bundle By Name(cluster=w457, "high limit (10V)"=w453, "low limit (-10V)"=w454, "Ch No"=w455, "Var name"=w459) -> (w452:T11)
                    n128 = Build Array (concatenate)(w452, w451) -> (w460:T13)
                  }
                }
              }
              frame 1.. {
                n129 = Unbundle By Name(w464) -> ("high limit (10V)"=w470:sgl, "low limit (-10V)"=w469:sgl, "Ch No"=w468:i16, "Calib filename"=w466:path)
                n130 = Bundle By Name(cluster=w465, "high limit (10V)"=w470, "low limit (-10V)"=w469, "Ch No"=w468, "Var name"=w463) -> (w462:T11)
                n131 = local write "Type"(w462) -> ()
                n132 = Build Array (concatenate)(w462, w461) -> (w467:T13)
              }
            }
          }
          frame #10 {
            n133 = case shown="True" "Edit temp and Press" {
              frame False {
              }
              frame True {
                n134 = stacked-sequence {
                  frame #0 {
                    w472 = TRUE  # Wait until done
                    n135 = call "Run_Enter_Temp.vi"("Wait until done"=w472) -> ()  [unwired: 1 out]
                  }
                  frame #1 {
                    n136 = call "Get_Temp_and_Press.vi"("Averaging time (mins)"=0.5) -> ("Abs Press (mbar)"=w474:dbl, "Temperature"=w473:dbl)  [unwired: 3 out]
                    n137 = local write "Abs Press (mbar)"(w474) -> ()
                    n138 = local write "Temp (deg C)"(w473) -> ()
                  }
                }
              }
            }
          }
          frame #11 {
            n139 = case shown="False" "OK" {
              tunnel: w478 -> [_ w482]
              tunnel: [TRUE w481] -> w476
              frame False {
              }
              frame True {
                n140 = stacked-sequence {
                  seq-local: [w483 _] -> [_ w501]
                  tunnel: w482 -> [w485 w503]
                  tunnel: [_ w499] -> w481
                  frame #0 {
                    n141 = for {
                      shift-right: [w492] -> _
                      shift-left: i16[] [] -> [w491]
                      tunnel: w485 -> [w488] mode=indexing
                      tunnel: [w487] -> w484 mode=indexing
                      n142 = Unbundle By Name(w488) -> ("Ch No"=w489:i16)
                      n143 = Search 1D Array(1D array=w491, element=w489) -> (index of element=w490:i32)  [unwired: 1 out]
                      n144 = Build Array (concatenate)(w491, w489) -> (w492:i16[])
                      n145 = case shown="0, Default" w490 {
                        tunnel: w489 -> [w497 _]
                        tunnel: [w493 FALSE ("true")] -> w487
                        frame 0, Default {
                          n146 = Format Into String(format string="The Ch No %d appears more than once", w497) -> (resulting string=w495:string)  [unwired: 2 in, 1 out]
                          n147 = One Button Dialog(message=w495, button name ("OK")="Ok") -> (true=w493:bool)
                        }
                        frame -1 {
                        }
                      }
                    }
                    n148 = Or Array Elements(Boolean array=w484) -> (logical OR=w483:bool)
                  }
                  frame #1 {
                    n149 = for {
                      tunnel: w503 -> [w509] mode=indexing
                      tunnel: [w508] -> w502 mode=indexing
                      n150 = Unbundle By Name(w509) -> ("high limit (10V)"=w507:sgl, "low limit (-10V)"=w506:sgl, "Ch No"=w504:i16)
                      n151 = Greater Or Equal?(x=w507, y=w506) -> (x >= y?=w505:bool)
                      n152 = case shown="False" w505 {
                        tunnel: [TRUE ("true") FALSE ("true")] -> w508
                        tunnel: w504 -> [w511 _]
                        frame False {
                          n153 = Number To Decimal String(number=w511) -> (decimal integer string=w512:string)  [unwired: 1 out]
                          n154 = Concatenate Strings("Error in input limits for Channel No ", w512) -> (w513:string)
                          n155 = One Button Dialog(message=w513) -> ()  [unwired: 2 out]
                        }
                        frame True {
                        }
                      }
                    }
                    n156 = Or Array Elements(Boolean array=w502) -> (logical OR=w500:bool)
                    n157 = Or(x=w500, y=w501) -> (x .or. y?=w499:bool)
                  }
                }
              }
            }
          }
          frame #12 {
            n158 = Unbundle By Name(w519) -> ("Ref Instrument type"=w518:T2)
            n159 = Equal?(x=Ref_Inst_type."Preston tube" ("Ref Instrument type"), y=w518) -> (x = y?=w516:bool)
            n160 = property on="Preston tube diammeter in mm" class="DigNum (strict)"("Visible"=w516) -> ()  [unwired: 2 in, 2 out]
          }
        }
      }
      "Instrument type" <- w71
      "Ch & spans" <- w74
      "Calib filename" <- w73
      n161 = global write "Calib_global.vi" "Angle/vel calib file"(w67) -> ()
      n162 = global write "Calib_global.vi" "existing angle calib"(w66) -> ()
    }
    frame #4 {
      n163 = global read "Calib_global.vi" "Pre Setup String"() -> (w521:string)
      n164 = case shown="\"Setup Front Panel\"" w526 {
        tunnel: [w528 w538] -> w525
        tunnel: "Sampling speeds" -> [w528 w540]
        tunnel: [w527 w534] -> w523
        tunnel: "Fixed n" -> [w527 _]
        tunnel: w521 -> [_ w533]
        tunnel: w520 -> [_ _]
        frame "Show Setup", Default {
        }
        frame "Setup Front Panel" {
          n165 = call "Get_value_from_string.vi"("Input string"=w533, "Variable name"="Requested sampling rate") -> ("Status"=w531:enum16{"Char in string", "Char not in string"}, "Value"=w529:dbl)  [unwired: 1 in]
          n166 = case shown="\"Char not in string\"" w531 {
            tunnel: [w542 sgl 100.0 ("Sampling Rate /ch (Hz)")] -> w530
            tunnel: w529 -> [w542 _]
            frame "Char in string" {
            }
            frame "Char not in string" {
            }
          }
          n167 = call "Get_value_from_string.vi"("Input string"=w533, "Variable name"="No of samples") -> ("Value"=w539:dbl)  [unwired: 1 in, 1 out]
          n168 = call "Get_Characters_from_string.vi"("Input string"=w533, "Variable name"="Fixed Coefficient n") -> ("Value"=w536:string)  [unwired: 1 in, 1 out]
          n169 = Bundle By Name(cluster=w540, "Samples /ch"=w539, "Sampling Rate /ch (Hz)"=w530) -> (w538:T5)
          n170 = Equal?(x="TRUE", y=w536) -> (x = y?=w534:bool)
        }
      }
      "Sampling speeds Output" <- w525
      "Fixed n out" <- w523
    }
    frame #5 {
      n171 = property on="Calib filename" class="Path"() -> ("Disabled"=w548:u8)  [unwired: 2 in, 2 out]
      n172 = Equal To 0?(x=w548) -> (x = 0?=w547:bool)
      n173 = local read "Reference instrument"() -> (w546:T7)
      n174 = case shown="True" w547 {
        tunnel: w546 -> [w551 w557]
        tunnel: [w550 w556] -> w545
        tunnel: w544 -> [_ w552]
        frame False {
          n175 = Bundle By Name(cluster=w551, "Calib filename"=path "") -> (w550:T7)
        }
        frame True {
          w553 = FALSE  # Use Latest Calib
          n176 = Unbundle By Name(w557) -> ("Calib filename"=w559:path, "Ref Instrument type"=w555:T2)
          n177 = case shown="\"ADAM Channel\"" w555 {
            tunnel: [Inst_type."Propeller anemometer" ("Inst type") Inst_type."Pressure Transducer" ("Inst type") Inst_type."Pressure Transducer" ("Inst type") Inst_type."Pitot-static tube" ("Inst type") Inst_type."Preston tube" ("Inst type") Inst_type."Generic Linear" ("Inst type") Inst_type."Generic Polynomial" ("Inst type") Inst_type."Thermocouple" ("Inst type") Inst_type."Raw voltage" ("Inst type") Inst_type."Raw voltage" ("Inst type") Inst_type."Raw voltage" ("Inst type")] -> w554
            frame "Propellor anemometer" {
            }
            frame "Pressure Transducer" {
            }
            frame "Raw voltage" {
            }
            frame "Pitot-static tube" {
            }
            frame "Preston tube" {
            }
            frame "Generic Linear" {
            }
            frame "Generic Polynomial" {
            }
            frame "Thermocouple" {
            }
            frame "LDA" {
            }
            frame "Enter Value" {
            }
            frame "ADAM Channel" {
            }
          }
          n178 = case shown="\"Take a New Calibration Point\", Default" w552 {
            tunnel: w559 -> [w560 w564]
            tunnel: [w560 w563] -> w558
            tunnel: w554 -> [_ w562]
            tunnel: w553 -> [_ w561]
            frame "Refit Curve" {
            }
            frame "Take a New Calibration Point", Default {
              n179 = call "Find_calibration_file.vi"("Inst type"=w562, "Use Latest Calib"=w561, "filename"=w564) -> ("filename out"=w563:path)  [unwired: 1 in]
            }
          }
          n180 = Bundle By Name(cluster=w557, "Calib filename"=w558) -> (w556:T7)
        }
      }
      n181 = local write "Reference instrument"(w545) -> ()
    }
    frame #6 {
      n182 = property on="Ref vel for angle calib" class="Clust (strict)"() -> ("Disabled"=w576:u8)  [unwired: 2 in, 2 out]
      n183 = local read "Ref vel for angle calib"() -> (w578:T7)
      n184 = case shown="0" w576 {
        tunnel: w578 -> [w583 w599]
        tunnel: [w582 w598] -> w577
        frame 0 {
          w579 = FALSE  # Use Latest Calib
          n185 = Unbundle By Name(w583) -> ("Calib filename"=w585:path, "Ref Instrument type"=w581:T2)
          n186 = case shown="\"Preston tube\"" w581 {
            tunnel: [Inst_type."Propeller anemometer" ("Inst type") Inst_type."Pressure Transducer" ("Inst type") Inst_type."Pressure Transducer" ("Inst type") Inst_type."Pitot-static tube" ("Inst type") Inst_type."Preston tube" ("Inst type") Inst_type."Generic Linear" ("Inst type") Inst_type."Generic Polynomial" ("Inst type") Inst_type."Thermocouple" ("Inst type") Inst_type."Raw voltage" ("Inst type") Inst_type."Raw voltage" ("Inst type") Inst_type."Raw voltage" ("Inst type")] -> w580
            frame "Propellor anemometer" {
            }
            frame "Pressure Transducer" {
            }
            frame "Raw voltage" {
            }
            frame "Pitot-static tube" {
            }
            frame "Preston tube" {
            }
            frame "Generic Linear" {
            }
            frame "Generic Polynomial" {
            }
            frame "Thermocouple" {
            }
            frame "LDA" {
            }
            frame "Enter Value" {
            }
            frame "ADAM Channel" {
            }
          }
          n187 = call "Find_calibration_file.vi"("Inst type"=w580, "Use Latest Calib"=w579, "filename"=w585) -> ("filename out"=w584:path)  [unwired: 1 in]
          n188 = Bundle By Name(cluster=w583, "Calib filename"=w584) -> (w582:T7)
        }
        frame 1, Default {
          n189 = Bundle By Name(cluster=w599, "Calib filename"=path "") -> (w598:T7)
        }
      }
      n190 = local write "Ref vel for angle calib"(w577) -> ()
    }
    frame #7 {
      w606 = Ref_Inst_type."ADAM Channel" ("Ref Instrument type")
      n191 = local read "Ref vel for angle calib"() -> (w608:T7)
      n192 = global write "Calib_global.vi" "Ref Instrument type"(w603) -> ()
      n193 = property on="Ref vel for angle calib" class="Clust (strict)"() -> ("Disabled"=w601:u8)  [unwired: 2 in, 2 out]
      n194 = Unbundle By Name(w608) -> ("Ref Instrument type"=w607:T2)
      n195 = Equal To 0?(x=w601) -> (x = 0?=w600:bool)
      n196 = Equal?(x=w603, y=w606) -> (x = y?=w605:bool)
      n197 = local read "2nd ref instrument"() -> (w609:T6)
      n198 = Bundle By Name(cluster=w609, "2nd Ref type"=w607, "2nd inst present"=w600) -> (→"2nd ref instrument":T6)
      n199 = case shown="True" w600 {
        tunnel: w607 -> [_ w615]
        tunnel: w606 -> [_ w614]
        tunnel: w605 -> [w610 w612]
        tunnel: [w610 w611] -> w604
        frame False {
        }
        frame True {
          n200 = Equal?(x=w615, y=w614) -> (x = y?=w613:bool)
          n201 = Or(x=w613, y=w612) -> (x .or. y?=w611:bool)
        }
      }
    }
    frame #8 {
      n202 = Equal?(x=Calib_mode."Show Setup" ("Mode"), y=w623) -> (x = y?=w622:bool)
      n203 = And(x=w622, y=w621) -> (x .and. y?=w620:bool)
      n204 = global read "Calib_global.vi" "Pre Setup String"() -> (w619:string)
      n205 = case shown="True" w620 {
        tunnel: [w626 w632] -> w624
        tunnel: w619 -> [w628 w631]
        tunnel: "ADAM Channel name" -> [w627 w630]
        tunnel: [w625 w629] -> w617
        frame False {
          n206 = call "Get_Characters_from_string.vi"("Input string"=w628, "Variable name"=w627) -> ("Value"=w625:string)  [unwired: 1 in, 1 out]
          n207 = call "Characters_to_string.vi"("Characters to write"=w625, "Label for characters"=w627) -> ("Output string"=w626:string)
        }
        frame True {
          n208 = stacked-sequence {
            seq-local: [_ w636 _ _ _ _] -> [_ _ _ w646 _ _]
            seq-local: [_ _ _ w640 _ _] -> [_ _ _ _ _ _]
            seq-local: [_ _ w638 _ _ _] -> [_ _ _ _ _ w656]
            tunnel: [_ _ _ _ _ w655] -> w632
            tunnel: w631 -> [_ _ _ _ _ w651]
            tunnel: w630 -> [_ _ _ _ _ w650]
            tunnel: [_ _ _ _ _ w649] -> w629
            frame #0 {
              n209 = property on="Message" class="Str"("Visible"=TRUE) -> ()  [unwired: 2 in, 2 out]
              "Message" <- "Message\n\nCurrently trying to connect to the server.\n\nPlease Wait"
            }
            frame #1 {
              n210 = Get Date/Time In Seconds() -> (seconds since 1Jan1904=w635:timestamp)
              n211 = To Double Precision Float(number=w635) -> (double precision float=w636:dbl)
            }
            frame #2 {
              n212 = call "Get_ADAM_Ch_names_client.vi"("Channel names set"=Channel_names."Active Only") -> ("Ch names"=w638:string[])
            }
            frame #3 {
              n213 = Get Date/Time In Seconds() -> (seconds since 1Jan1904=w639:timestamp)
              n214 = To Double Precision Float(number=w639) -> (double precision float=w645:dbl)
              n215 = Subtract(x=w645, y=w646) -> (x-y=w644:dbl)
              n216 = Number To Decimal String(number=w644) -> (decimal integer string=w642:string)  [unwired: 1 out]
              n217 = Concatenate Strings("Server took ", w642, " Seconds to respond") -> (w640:string)
            }
            frame #4 {
              n218 = property on="Message" class="Str"("Visible"=FALSE) -> ()  [unwired: 2 in, 2 out]
            }
            frame #5 {
              n219 = call "Get_Characters_from_string.vi"("Input string"=w651, "Variable name"=w650) -> ("Status"=w654:enum16{"Char in string", "Char not in string"}, "Value"=w653:string)  [unwired: 1 in]
              n220 = case shown="\"Char in string\"" w654 {
                tunnel: w653 -> [w657 _]
                tunnel: [w657 "" ("Value")] -> w652
                frame "Char in string" {
                }
                frame "Char not in string" {
                }
              }
              n221 = call "Select_Single_ADAM_Ch.vi"("Desired Ch name (in)"=w652, "Available Ch names"=w656, "Message"="Please Choose Reference Instrument") -> ("Ch Name"=w649:string)  [unwired: 3 out]
              n222 = call "Characters_to_string.vi"("Characters to write"=w649, "Label for characters"=w650) -> ("Output string"=w655:string)
            }
          }
        }
      }
      n223 = global write "Calib_global.vi" "ADAM Channel Name"(w617) -> ()
    }
    frame #9 {
      n224 = local read "2nd ref instrument"() -> (w665:T6)
      n225 = Equal?(x=Calib_mode."Show Setup" ("Mode"), y=w672) -> (x = y?=w671:bool)
      n226 = Unbundle By Name(w665) -> ("2nd Ref type"=w663:T2, "2nd inst present"=w661:bool)
      n227 = global read "Calib_global.vi" "Pre Setup String"() -> (w669:string)
      n228 = Equal?(x=Ref_Inst_type."ADAM Channel" ("2nd Ref type"), y=w663) -> (x = y?=w662:bool)
      n229 = And(x=w662, y=w661) -> (x .and. y?=w660:bool)
      n230 = And(x=w671, y=w660) -> (x .and. y?=w670:bool)
      n231 = case shown="True" w670 {
        tunnel: [w674 w680] -> w659
        tunnel: w669 -> [w676 w679]
        tunnel: "ADAM Channel name for 2nd Ref Instr" -> [w675 w678]
        tunnel: [w673 w677] -> w667
        frame False {
          n232 = call "Get_Characters_from_string.vi"("Input string"=w676, "Variable name"=w675) -> ("Value"=w673:string)  [unwired: 1 in, 1 out]
          n233 = call "Characters_to_string.vi"("Characters to write"=w673, "Label for characters"=w675) -> ("Output string"=w674:string)
        }
        frame True {
          n234 = stacked-sequence {
            seq-local: [_ w684 _ _ _ _] -> [_ _ _ w694 _ _]
            seq-local: [_ _ _ w688 _ _] -> [_ _ _ _ _ _]
            seq-local: [_ _ w686 _ _ _] -> [_ _ _ _ _ w704]
            tunnel: [_ _ _ _ _ w703] -> w680
            tunnel: w679 -> [_ _ _ _ _ w699]
            tunnel: w678 -> [_ _ _ _ _ w698]
            tunnel: [_ _ _ _ _ w697] -> w677
            frame #0 {
              n235 = local write "Message"("Message\n\nCurrently trying to connect to the server.\n\nPlease Wait") -> ()
              n236 = property on="Message" class="Str"("Visible"=TRUE) -> ()  [unwired: 2 in, 2 out]
            }
            frame #1 {
              n237 = Get Date/Time In Seconds() -> (seconds since 1Jan1904=w683:timestamp)
              n238 = To Double Precision Float(number=w683) -> (double precision float=w684:dbl)
            }
            frame #2 {
              n239 = call "Get_ADAM_Ch_names_client.vi"("Channel names set"=Channel_names."Active Only") -> ("Ch names"=w686:string[])
            }
            frame #3 {
              n240 = Get Date/Time In Seconds() -> (seconds since 1Jan1904=w687:timestamp)
              n241 = To Double Precision Float(number=w687) -> (double precision float=w693:dbl)
              n242 = Subtract(x=w693, y=w694) -> (x-y=w692:dbl)
              n243 = Number To Decimal String(number=w692) -> (decimal integer string=w690:string)  [unwired: 1 out]
              n244 = Concatenate Strings("Server took ", w690, " Seconds to respond") -> (w688:string)
            }
            frame #4 {
              n245 = property on="Message" class="Str"("Visible"=FALSE) -> ()  [unwired: 2 in, 2 out]
            }
            frame #5 {
              n246 = call "Get_Characters_from_string.vi"("Input string"=w699, "Variable name"=w698) -> ("Status"=w702:enum16{"Char in string", "Char not in string"}, "Value"=w701:string)  [unwired: 1 in]
              n247 = case shown="\"Char in string\"" w702 {
                tunnel: w701 -> [w705 _]
                tunnel: [w705 "" ("Value")] -> w700
                frame "Char in string" {
                }
                frame "Char not in string" {
                }
              }
              n248 = call "Select_Single_ADAM_Ch.vi"("Desired Ch name (in)"=w700, "Available Ch names"=w704, "Message"="Please Choose 2nd Ref Channel") -> ("Ch Name"=w697:string)  [unwired: 3 out]
              n249 = call "Characters_to_string.vi"("Characters to write"=w697, "Label for characters"=w698) -> ("Output string"=w703:string)
            }
          }
        }
      }
      n250 = global write "Calib_global.vi" "ADAM Channel Name Vel Ref"(w667) -> ()
    }
    frame #10 {
      n251 = local read "Reference instrument"() -> (w711:T7)
      n252 = local read "2nd ref instrument"() -> (w712:T6)
      n253 = local read "Sampling speeds Output"() -> (w708:T5)
      n254 = local read "Abs Press (mbar)"() -> (w709:dbl)
      n255 = global write "Calib_global.vi" "2nd ref instrument"(w712) -> ()
      n256 = local read "Temp (deg C)"() -> (w707:dbl)
      n257 = Unbundle By Name(w708) -> ("Sampling Rate /ch (Hz)"=w714:sgl, "Samples /ch"=w715:i32)
      n258 = global write "Calib_global.vi" "Abs Press (mbar)"(w709) -> ()
      n259 = global write "Calib_global.vi" "Temp (deg C)"(w707) -> ()
      n260 = call "Calib_General_Setup.vi"("Reference instrument"=w711, "Requested No of samples"=w715, "Sampling rate (Hz)"=w714, "2nd ref instrument"=w712, "Temp"=w707, "Board type"=w716, "Abs Press (mbar)"=w709) -> ("Output string"=w713:string, "LDA Data"=w710:bool)  [unwired: 7 out]
      n261 = global write "Meas_global.vi" "Board type"(w716) -> ()
    }
    frame #11 {
      n262 = local read "Ref vel for angle calib"() -> (w725:T7)
      n263 = local read "Reference instrument"() -> (w724:T7)
      n264 = local read "Instrument type"() -> (w723:T8)
      n265 = global write "Calib_global.vi" "Instrument type"(w723) -> ()
      n266 = case shown="\"Propeller anemometer\", Default" w723 {
        tunnel: [w728 w729 w731] -> w722
        tunnel: w725 -> [w727 w730 _]
        tunnel: [w727 w730 w731] -> w718
        tunnel: w724 -> [w728 w729 w731]
        frame "Propeller anemometer", Default {
        }
        frame "Cross wire angle" {
        }
        frame "Cross wire velocity" {
        }
      }
      n267 = call "Reference_Inst_Info_2_string.vi"("Reference instrument"=w722, "Reference Name"="Reference instrument") -> ("Setup String"=w720:string)
      n268 = call "Reference_Inst_Info_2_string.vi"("Reference instrument"=w718, "Reference Name"="Ref vel for angle calib") -> ("Setup String"=w717:string)
      n269 = Concatenate Strings(w720, w717) -> (w726:string)
    }
    frame #12 {
      n270 = local read "Instrument type"() -> (w732:T8)
      n271 = case shown="\"Pulsed Wire\"" w732 {
        tunnel: ["" w741] -> w733
        tunnel: w734 -> [_ w740]
        frame "Propeller anemometer", Default {
        }
        frame "Pulsed Wire" {
          w736 = FALSE  # Check Calib file?
          n272 = case shown="\"Refit Curve\", Default" w740 {
            tunnel: [w743 w745] -> w739
            tunnel: [w742 w744] -> w738
            frame "Refit Curve", Default {
              w743 = FALSE  # Show Panel?
              w742 = T14 TRUE  # OK
            }
            frame "Show Setup" {
              w745 = TRUE  # Show Panel?
              w744 = T14 FALSE  # OK
            }
          }
          n273 = global read "Calib_global.vi" "Pre Setup String"() -> (w737:string)
          n274 = call "PWA_Setup_Panel.vi"("Show Panel?"=w739, "Check Calib file?"=w736, "OK"=w738, "Incoming Setup String"=w737) -> ("Outgoing Setup String"=w741:string)  [unwired: 3 out]
        }
      }
    }
    frame #13 {
      n275 = local read "instrument to calibrate"() -> (w748:T10)
      n276 = for {
        tunnel: w748 -> [w775] mode=indexing
        shift-right: [w760] -> w751
        shift-left: "" -> [w764]
        i -> [w774]
        n277 = Unbundle By Name(w775) -> ("high limit (10V)"=w771:sgl, "low limit (-10V)"=w766:sgl, "Ch No"=w765:i16)
        n278 = Increment(x=w774) -> (x+1=w759:i32)
        n279 = Format Into String(format string="Inst_to_calibrate_element_%d ", w759) -> (resulting string=w757:string)  [unwired: 2 in, 1 out]
        n280 = Concatenate Strings(w757, "Low limit") -> (w770:string)
        n281 = Concatenate Strings(w757, "Ch No") -> (w769:string)
        n282 = Concatenate Strings(w757, "High limit") -> (w772:string)
        n283 = call "Value_to_string.vi"("Value"=w766, "Label for value"=w770) -> ("Output string"=w762:string)  [unwired: 1 in]
        n284 = call "Value_to_string.vi"("Value"=w765, "Label for value"=w769) -> ("Output string"=w761:string)  [unwired: 1 in]
        n285 = call "Value_to_string.vi"("Value"=w771, "Label for value"=w772) -> ("Output string"=w763:string)  [unwired: 1 in]
        n286 = Concatenate Strings(w764, w763, w762, w761) -> (w760:string)
      }
      n287 = Array Size(array=w748) -> (size(s)=w747:i32)
      n288 = Equal To 0?(x=w747) -> (x = 0?=w746:bool)
      n289 = case shown="True" w746 {
        tunnel: [w753 i16 -10 ("Ch No")] -> w749
        tunnel: w748 -> [w752 _]
        frame False {
          w755 = 0  # index
          n290 = Index Array(array=w752, index=w755) -> (element=w754:T19)
          n291 = Unbundle By Name(w754) -> ("Ch No"=w753:i16)
        }
        frame True {
        }
      }
      n292 = global write "Calib_global.vi" "Calib Ch No"(w749) -> ()
    }
    frame #14 {
      n293 = local read "Preston tube diammeter in mm"() -> (w779:dbl)
      n294 = local read "Instrument type"() -> (w790:T8)
      n295 = property on="Instrument type" class="Enum (strict)"() -> ("Strings []"=w791:string[])  [unwired: 2 in, 2 out]
      n296 = local read "angle calib"() -> (w784:T9)
      n297 = property on="angle calib" class="Enum (strict)"() -> ("Strings []"=w785:string[])  [unwired: 2 in, 2 out]
      n298 = Index Array(array=w791, index=w790) -> (element=w789:string)
      n299 = Index Array(array=w785, index=w784) -> (element=w783:string)
      n300 = call "Characters_to_string.vi"("Characters to write"=w789, "Label for characters"="Instrument_type_to Calibrate") -> ("Output string"=w787:string)
      n301 = call "Value_to_string.vi"("Value"=w779, "Label for value"="Preston tube diameter in mm" ("Variable name")) -> ("Output string"=w778:string)  [unwired: 1 in]
      n302 = call "Characters_to_string.vi"("Characters to write"=w783, "Label for characters"="Angle calib") -> ("Output string"=w782:string)
      n303 = local read "Fixed n out"() -> (w795:bool)
      n304 = Concatenate Strings(w778, w787, w782) -> (w802:string)
      n305 = Select(t="TRUE", s=w795, f="FALSE") -> (s? t:f=w796:string)
      n306 = global read "Calib_global.vi" "New Setup String"() -> (w794:string)
      n307 = call "Characters_to_string.vi"("Characters to write"=w796, "Label for characters"="Fixed Coefficient n") -> ("Output string"=w792:string)
      n308 = Concatenate Strings(w794, w792, w802, w801, w776, w800, w777, w793, w781) -> (w803:string)
      n309 = global write "Calib_global.vi" "New Setup String"(w803) -> ()
    }
    frame #15 {
      n310 = Equal?(x=Calib_mode."Show Setup" ("Mode"), y=w809) -> (x = y?=w808:bool)
      n311 = And(x=w807, y=w808) -> (x .and. y?=w806:bool)
      n312 = case shown="True" w806 {
        tunnel: [FALSE ("Synchronise with LDA") FALSE ("Synchronise with LDA")] -> w804
        frame False {
        }
        frame True {
          n313 = global read "LDA_meas_global_1.vi" "BSA Type"() -> (w813:T20)
          n314 = case shown="\"57N11\"" w813 {
            tunnel: TRUE -> [_ w820]
            frame "57N11" {
              n315 = stacked-sequence {
                frame #0 {
                  n316 = global write "Meas_global.vi" "dimensions"(enum16{"1D", "2D"}."1D" ("dimensions")) -> ()
                }
                frame #1 {
                  w815 = "1"  # BSA Number
                  n317 = call "Control_BSA_setup.vi"("setup"=Setup."Show Setup", "BSA number"=w815) -> ()  [unwired: 14 out]
                }
                frame #2 {
                  n318 = global read "LDA_meas_global_2.vi" "BSA2 info"() -> (w817:T21)
                  n319 = Unbundle By Name(w817) -> ("GPIB Address"=w818:string)
                  n320 = call "Set_BSA_Coincidence.vi"("GPIB address"=w818, "Set Coincidence"=enum16{"Slave", "Master", "Private"}."Slave") -> ()  [unwired: 1 in, 5 out]
                }
              }
            }
            frame "BSA F60" {
              n321 = disable-structure shown="TARGET_TYPE==Windows" {
                disable-tunnel: w820 -> [_ w821]
                frame condition #0 (active) {
                }
                frame condition #1 {
                  n322 = call "Edit_BSA_IP.vi"("Show Panel"=w821) -> ()  [unwired: 3 out]
                }
              }
            }
          }
        }
      }
      n323 = global write "Meas_global.vi" "Synchronise with LDA"(w804) -> ()
    }
    frame #16 {
      w829 = TRUE  # Lock File
      w839 = FALSE  # advisory dialog? (display:T)
      w840 = FALSE  # append to file? (new file:F)
      n324 = local read "Instrument type"() -> (w827:T8)
      n325 = local read "Calib filename"() -> (w841:path)
      n326 = global read "Meas_global.vi" "LDA data"() -> (w832:enum16{"No LDA data", "Take LDA data"})
      n327 = global write "Calib_global.vi" "Ref Calib file"(w841) -> ()
      n328 = local read "Ch & spans"() -> (w833:T13)
      n329 = case shown="\"Take LDA data\"" w832 {
        tunnel: ["" w849] -> w830
        frame "No LDA data" {
        }
        frame "Take LDA data" {
          n330 = call "LDA_header.vi"() -> ("LDA Header string"=w851:string)  [unwired: 3 out]
          n331 = call "LDA_U16_data_header.vi"() -> ("Output string"=w850:string)  [unwired: 1 out]
          n332 = Concatenate Strings(w851, w850) -> (w849:string)
        }
      }
      n333 = case shown="\"Pulsed Wire\"" w827 {
        tunnel: ["" w843] -> w826
        frame "Propeller anemometer", Default {
        }
        frame "Pulsed Wire" {
          n334 = property on="PWA Data" class="Enum (strict)"() -> ("Strings []"=w846:string[])  [unwired: 2 in, 2 out]
          n335 = Index Array(array=w846, index=PWA_Data."One Ch PWA" ("PWA Data")) -> (element=w844:string)
          n336 = call "Characters_to_string.vi"("Characters to write"=w844, "Label for characters"="Pulsed_Wire_Data" ("Variable name")) -> ("Output string"=w843:string)
        }
      }
      n337 = call "Calib_Ch_setup.vi"("Preston tube diammeter in mm"="Preston tube diammeter in mm", "Ch & spans"=w833, "Calib filename"=w841) -> ("Output string"=w834:string)
      n338 = global write "Calib_global.vi" "Ch & spans"(w833) -> ()
      n339 = call "Date_and_Time_to_string.vi"() -> ("Date and time (spreadsheet)"=w831:string)
      n340 = Concatenate Strings(w831, w826, w830, w835, w834, w825) -> (w836:string)
      n341 = call "Setup_Filepath.vi"("Setup File Type"=Setup_Filetype."Measurement Setups", "Filename in"="Calib_Setup.xls") -> ("Filename Out"=w822:path)  [unwired: 1 out]
      n342 = call "Add_label_to_string.vi"("String to write"=w836, "File Label"="Raw data header") -> ("Output string"=w837:string)
      n343 = call "Write_Characters_To_File.vi"("file path (dialog if empty)"=w822, "advisory dialog? (display:T)"=w839, "character string"=w837, "append to file? (new file:F)"=w840, "Lock File"=w829) -> ()  [unwired: 4 out]
    }
    frame #17 {
      n344 = case shown="\"Show Setup\"" w852 {
        frame "Show Setup" {
          n345 = Current VI's Path() -> (path=w854:path)
          n346 = call "Open_Close_Front_Panel.ph.vi"("Front Panel Window:Open"=FALSE, "VI path"=w854) -> ()  [unwired: 2 out]
        }
        frame "Take a New Calibration Point", Default {
        }
      }
    }
  }
